vi "Taiko_UpdateTaggedValueList.vi"(9 "TaggedValueList all":T1 {"Tag" format="%x" items=["NONE"=0, "Locked"=16, "SoftLock"=17, "KeyLock"=18, "Class_IV_Lock"=20, "Interlock"=24, "LaserMode"=32, "LDH_PulsePowerTable"=33, "TriggerMode"=48, "TriggerLevelRaw"=64, "TriggerLevelRawLoLimit"=65, "TriggerLevelRawHiLimit"=66, "TriggerLevel"=72, "TriggerLevelLoLimit"=73, "TriggerLevelHiLimit"=74, "FastGate"=80, "FastGateImp"=96, "SlowGate"=112, "TargetTempRaw"=144, "TargetTempRawLoLimit"=145, "TargetTempRawHiLimit"=146, "CurrentTempRaw"=148, "CaseTempRaw"=149, "TargetTemp"=152, "TargetTempLoLimit"=153, "TargetTempHiLimit"=154, "CurrentTemp"=156, "CaseTemp"=157, "TempScale"=159, "Frequency"=168, "FrequencyLoLimit"=169, "FrequencyHiLimit"=170, "PulsePowerRaw"=176, "PulsePowerRawLoLimit"=177, "PulsePowerRawHiLimit"=178, "PulsePowerPermille"=180, "PulseShape"=181, "PulsePower"=184, "PulsePowerLoLimit"=185, "PulsePowerHiLimit"=186, "PulsePowerNanowatt"=188, "PulsePowerVoltage"=190, "PulseEnergy"=191, "CwPowerRaw"=192, "CwPowerRawLoLimit"=193, "CwPowerRawHiLimit"=194, "CwPowerPermille"=196, "CwPower"=200, "CwPowerLoLimit"=201, "CwPowerHiLimit"=202, "CwPowerMicroWatt"=204, "BurstLen"=208, "BurstPeriod"=224, "LDH_Fan"=240, "UI_Exclusive"=256]}, 10 "ListLen in":u32, 11 "TaggedValueList in":T1 {"Tag" format="%x" items=["NONE"=0, "Locked"=16, "SoftLock"=17, "KeyLock"=18, "Class_IV_Lock"=20, "Interlock"=24, "LaserMode"=32, "LDH_PulsePowerTable"=33, "TriggerMode"=48, "TriggerLevelRaw"=64, "TriggerLevelRawLoLimit"=65, "TriggerLevelRawHiLimit"=66, "TriggerLevel"=72, "TriggerLevelLoLimit"=73, "TriggerLevelHiLimit"=74, "FastGate"=80, "FastGateImp"=96, "SlowGate"=112, "TargetTempRaw"=144, "TargetTempRawLoLimit"=145, "TargetTempRawHiLimit"=146, "CurrentTempRaw"=148, "CaseTempRaw"=149, "TargetTemp"=152, "TargetTempLoLimit"=153, "TargetTempHiLimit"=154, "CurrentTemp"=156, "CaseTemp"=157, "TempScale"=159, "Frequency"=168, "FrequencyLoLimit"=169, "FrequencyHiLimit"=170, "PulsePowerRaw"=176, "PulsePowerRawLoLimit"=177, "PulsePowerRawHiLimit"=178, "PulsePowerPermille"=180, "PulseShape"=181, "PulsePower"=184, "PulsePowerLoLimit"=185, "PulsePowerHiLimit"=186, "PulsePowerNanowatt"=188, "PulsePowerVoltage"=190, "PulseEnergy"=191, "CwPowerRaw"=192, "CwPowerRawLoLimit"=193, "CwPowerRawHiLimit"=194, "CwPowerPermille"=196, "CwPower"=200, "CwPowerLoLimit"=201, "CwPowerHiLimit"=202, "CwPowerMicroWatt"=204, "BurstLen"=208, "BurstPeriod"=224, "LDH_Fan"=240, "UI_Exclusive"=256]}) -> (2 "Array":i32[](array[numeric]), 3 "TaggedValueList":T1 {"Tag" format="%x" items=["NONE"=0, "Locked"=16, "SoftLock"=17, "KeyLock"=18, "Class_IV_Lock"=20, "Interlock"=24, "LaserMode"=32, "LDH_PulsePowerTable"=33, "TriggerMode"=48, "TriggerLevelRaw"=64, "TriggerLevelRawLoLimit"=65, "TriggerLevelRawHiLimit"=66, "TriggerLevel"=72, "TriggerLevelLoLimit"=73, "TriggerLevelHiLimit"=74, "FastGate"=80, "FastGateImp"=96, "SlowGate"=112, "TargetTempRaw"=144, "TargetTempRawLoLimit"=145, "TargetTempRawHiLimit"=146, "CurrentTempRaw"=148, "CaseTempRaw"=149, "TargetTemp"=152, "TargetTempLoLimit"=153, "TargetTempHiLimit"=154, "CurrentTemp"=156, "CaseTemp"=157, "TempScale"=159, "Frequency"=168, "FrequencyLoLimit"=169, "FrequencyHiLimit"=170, "PulsePowerRaw"=176, "PulsePowerRawLoLimit"=177, "PulsePowerRawHiLimit"=178, "PulsePowerPermille"=180, "PulseShape"=181, "PulsePower"=184, "PulsePowerLoLimit"=185, "PulsePowerHiLimit"=186, "PulsePowerNanowatt"=188, "PulsePowerVoltage"=190, "PulseEnergy"=191, "CwPowerRaw"=192, "CwPowerRawLoLimit"=193, "CwPowerRawHiLimit"=194, "CwPowerPermille"=196, "CwPower"=200, "CwPowerLoLimit"=201, "CwPowerHiLimit"=202, "CwPowerMicroWatt"=204, "BurstLen"=208, "BurstPeriod"=224, "LDH_Fan"=240, "UI_Exclusive"=256]})   [LabVIEW 2010]
uses:
  _lib/PDLM/pdlm_lib_x86_x64_UIThread.llb/PDLM_Tag.ctl
  _lib/PDLM/pdlm_lib_x86_x64_UIThread.llb/PDLM_TaggedValue.ctl
  _lib/PDLM/pdlm_lib_x86_x64_UIThread.llb/PDLM_TaggedValueList.ctl
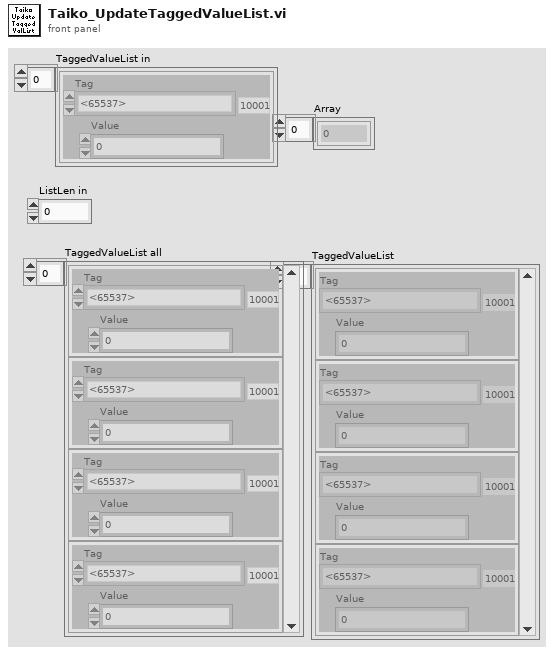
[diagram p1: front panel]
types:
  T1 = typedef "PDLM_TaggedValueList.ctl" = T2[]
  T2 = typedef "PDLM_TaggedValue.ctl" = cluster{"Tag":T3, "Value":u32}
  T3 = typedef "PDLM_Tag.ctl" = u32
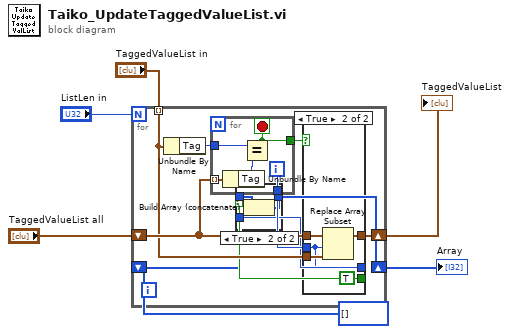
[diagram p0: block diagram]
diagram:
  n1 = for {
    N: "ListLen in" -> [_]
    tunnel: "TaggedValueList in" -> [w11] mode=indexing
    shift-right: [w13] -> w5
    shift-left: "TaggedValueList all" -> [w15]
    shift-right: [w7] -> w6
    shift-left: i32[] [] ("Array 2") -> [w8]
    n2 = Unbundle By Name(w11) -> ("Tag"=w16:T3)
    n3 = for {
      tunnel: w15 -> [w31] mode=indexing
      tunnel: w16 -> [w29]
      tunnel: [w28] -> w14
      tunnel: [w27] -> w12
      i -> [w28]
      stop <- w27 stop-if-true
      n4 = Unbundle By Name(w31) -> ("Tag"=w30:T3)
      n5 = Equal?(x=w29, y=w30) -> (x = y?=w27:bool)
    }
    n6 = case shown="True" w12 {
      tunnel: w15 -> [w21 w26]
      tunnel: w14 -> [_ w23]
      tunnel: [w21 w25] -> w13
      tunnel: w11 -> [_ w24]
      tunnel: [_ w23] -> w10
      tunnel: [_ TRUE] -> w9
      frame False {
      }
      frame True {
        n7 = Replace Array Subset(array=w26, new element=w24, index=w23) -> (w25:T1)
      }
    }
    n8 = case shown="True" w9 {
      tunnel: w8 -> [w17 w19]
      tunnel: w10 -> [_ w18]
      tunnel: [w17 w20] -> w7
      frame False {
      }
      frame True {
        n9 = Build Array (concatenate)(w19, w18) -> (w20:i32[])
      }
    }
  }
  "Array" <- w6
  "TaggedValueList" <- w5
